vi "Make_PSIMSSB_HIL.vi"(10 "Nu":dbl[](array[numeric])=[0.0, 0.0, 0.0]) -> (2 "PSIMSSB String":string)   [LabVIEW 2012]
panel:
  in  "Add info":dbl=0.4
  in  "Additional info (T = timelag)":string="T"
  in  "Expected Accuracy":dbl=0.7
  in  "SW filter (M = Measured)":string="M"
  in  "Orientation (N = North)":string="N"
  in  "Coord sys (C = Cartesian)":string="C"
  in  "Error Code (if status is V)":string
  in  "Status (A = OK, V = Error)":string="A"
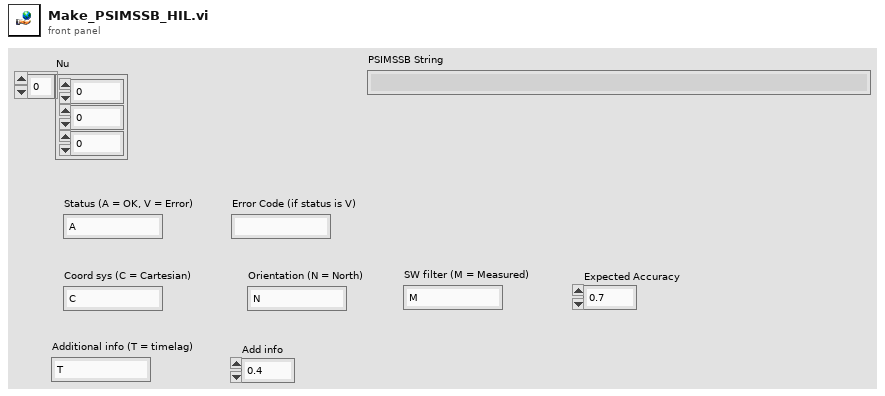
[diagram p1: front panel]
types:
  T1 = typedef "LVDateTimeRec.ctl" = cluster{"fractional second":dbl, "second":i32, "minute":i32, "hour":i32, "day of month":i32, "month":i32, "year":i32, "day of week":i32, "day of year":i32, "DST":i32}
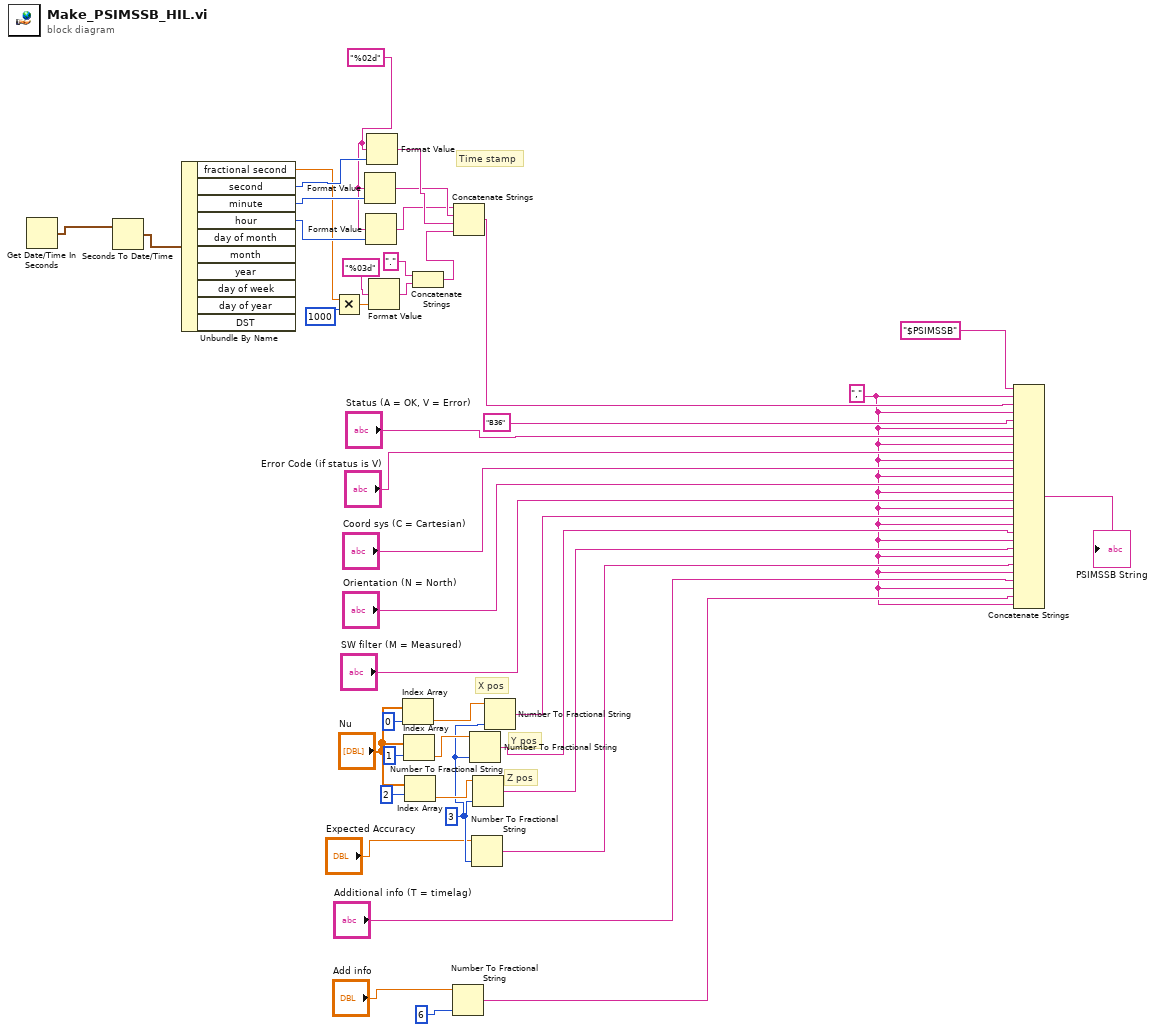
[diagram p0: block diagram]
diagram:
  w8 = 3
  w33 = "%02d"
  w1 = ","
  # "Z pos"
  # "Y pos"
  # "X pos"
  # "Time stamp"
  n1 = Get Date/Time In Seconds() -> (seconds since 1Jan1904=w41:timestamp)
  n2 = Seconds To Date/Time(time stamp (now)=w41) -> (date time rec=w40:T1)  [unwired: 1 in]
  n3 = Unbundle By Name(w40) -> ("fractional second"=w27:dbl, "second"=w39:i32, "minute"=w37:i32, "hour"=w36:i32)  [unwired: 6 out]
  n4 = Multiply(x=w27, y=1000) -> (x*y=w28:dbl)
  n5 = Format Value(format string=w33, value (0)=w37) -> (output string=w35:string)  [unwired: 1 in]
  n6 = Format Value(format string=w33, value (0)=w36) -> (output string=w34:string)  [unwired: 1 in]
  n7 = Format Value(format string=w33, value (0)=w39) -> (output string=w38:string)  [unwired: 1 in]
  n8 = Format Value(format string="%03d", value (0)=w28) -> (output string=w31:string)  [unwired: 1 in]
  n9 = Index Array(array="Nu", index=0) -> (element=w14:dbl)
  n10 = Index Array(array="Nu", index=1) -> (element=w13:dbl)
  n11 = Index Array(array="Nu", index=2) -> (element=w12:dbl)
  n12 = Concatenate Strings(".", w31) -> (w30:string)
  n13 = Number To Fractional String(number="Add info", precision (6)=6) -> (F-format string=w2:string)  [unwired: 2 in]
  n14 = Concatenate Strings(w34, w35, w38, w30) -> (w29:string)
  n15 = Number To Fractional String(number=w13, precision (6)=w8) -> (F-format string=w10:string)  [unwired: 2 in]
  n16 = Number To Fractional String(number="Expected Accuracy", precision (6)=w8) -> (F-format string=w6:string)  [unwired: 2 in]
  n17 = Number To Fractional String(number=w12, precision (6)=w8) -> (F-format string=w9:string)  [unwired: 2 in]
  n18 = Number To Fractional String(number=w14, precision (6)=w8) -> (F-format string=w11:string)  [unwired: 2 in]
  n19 = Concatenate Strings("$PSIMSSB", w1, w29, w1, "B36", w1, "Status (A = OK, V = Error)", w1, "Error Code (if status is V)", w1, "Coord sys (C = Cartesian)", w1, "Orientation (N = North)", w1, "SW filter (M = Measured)", w1, w11, w1, w10, w1, w9, w1, w6, w1, "Additional info (T = timelag)", w1, w2, w1) -> (→"PSIMSSB String":string)
